vi "Dashboard Main.vi"() -> ()   [LabVIEW 2014]
uses:
  <vilib>/event_ctls.llb/eventvkey.ctl
  <vilib>/Rock Robotics/WPI/Dashboard/WPI_DashboardLogging Global.vi
  <vilib>/Rock Robotics/Network Tables/SD Write Number.vi
  <vilib>/Rock Robotics/Network Tables/SD Write Boolean.vi
  <vilib>/Rock Robotics/Network Tables/SD Read Number.vi
  <vilib>/Rock Robotics/Network Tables/SD Read Boolean.vi
  <vilib>/Rock Robotics/Network Tables/SD Write String.vi
  <vilib>/Utility/config.llb/Write Key (String).vi
  <vilib>/Utility/config.llb/Write Key (I32).vi
  <vilib>/Utility/config.llb/NI_LVConfig.lvlib
panel:
  in  "TCP":refnum<k5>
  in  "Rec Mode":enum32{"Stop", "Record", "Playback"}(radio)
  in  "Vision":u16(ring) items=["Camera Off", "USB Camera SW", "USB Camera HW", "IP Camera"]
  out "Camera IP":string
  out "Image Message":string="Timeout in Camera Communications"
  in  "Dashboard Tab":T1(tab)
  out "?":bool
  in  "Motor Saftey":bool=TRUE
  in  "Camera Settings":T2={"Frame Rate"=30, "Compression"=30, "Size"=1} {"Frame Rate" scale=1.0..30.0; "Size" items=["640x480", "320x240", "160x120"]}
  out "MotorChart R":cluster{"Numeric":dbl, "Numeric":dbl}(graph)
  out "MotorChart L":T3(graph)
  out "MotorSliders R":cluster{"MotorSlide1":dbl, "MotorSlide2":dbl} {"MotorSlide2" scale=-1.0..1.0 scale format="%#_2e"; "MotorSlide1" scale=-1.0..1.0 scale format="%#_2e"}
  out "MotorSliders L":T4 {"MotorSlide4 2" scale=0.0..14.0 scale format="%#_2e"; "MotorSlide2" scale=-1.0..1.0 scale format="%#_2e"; "MotorSlide1" scale=-1.0..1.0 scale format="%#_2e"}
  out "Gyro":dbl(knob) scale=0.0..360.0
  out "JS1 Z":dbl(slide) scale=-1.0..1.0 scale format="%#_2e"
  out "JS1 Graph":cluster{"X":dbl, "Y":dbl}[](graph)
  out "JS1 Buttons":T5
  out "JS2 Z":dbl(slide) scale=-1.0..1.0 scale format="%#_2e"
  out "JS2 Graph":cluster{"X":dbl, "Y":dbl}[](graph)
  out "JS2 Buttons":T5
  out "Mode":T6(ring)=enum."Auto Disabled"
  in  "DB Camera Config":bool
  out "fps":dbl format="%#.1g"
  out "Mbps":dbl format="%#.1g"
  out "Mbps 2":bool
  in  "DB/String 9":string
  in  "DB/String 8":string
  in  "DB/String 7":string
  in  "DB/String 6":string
  in  "DB/String 5":string
  in  "DB/String 4":string
  in  "DB/String 3":string
  in  "DB/String 2":string
  in  "DB/String 1":string
  in  "DB/String 0":string
  in  "DB/Slider 0":dbl(slide) scale=0.0..5.0
  in  "DB/Slider 1":dbl(slide) scale=0.0..5.0
  in  "DB/Slider 2":dbl(slide) scale=0.0..5.0
  in  "DB/Slider 3":dbl(slide) scale=0.0..5.0
  out "DB/LED 3":bool
  out "DB/LED 2":bool
  out "DB/LED 1":bool
  out "DB/LED 0":bool
  in  "DB/Button 3":bool
  in  "DB/Button 2":bool
  in  "DB/Button 1":bool
  in  "DB/Button 0":bool caption="New Name"
  in  "Test Slider":dbl(slide) scale=0.0..100.0 scale format="%#_3g"
  in  "On/Off":bool caption="Solenoid"
  in  "Test Name":u16(ring) items=["Select the test to run...", "Example Test", "-------------------------------", "List of tests is built in robot code.", "Replace with your own automated tests."]
  in  "Test Tree":string(tree)
  in  "Motor":cluster{"Value":dbl, "Enable":bool} {"Value" scale=-1.0..1.0 scale format="%#_3g"}
  out "Progress":T7 {"Test Progress" scale=0.0..100.0}
  in  "Rev/Fwd":cluster{"Forward":bool, "Reverse":bool}
  in  "Test Ring":u16(ring) items=["Monochrome", "Color"]
  in  "Listbox":i32(listbox)
  in  "Autonomous Program":i32(listbox)
  in  "Test System Select":enum32{"Motors", "Pneumatics"}(tab)
  in  "Test Motor Mode Select":enum32{"Encoder Mode", "Manual Mode"}(tab)
  in  "?":bool
  in  "Motor Power":dbl(knob) scale=0.0..1.0
  out "?":bool=TRUE
  out "Encoder Feedback":dbl
  in  "Encoder Setpoint":dbl
  out "Encoder RPM":dbl
  in  "?":dbl(knob) scale=-1.0..1.0
  in  "Test Action":string(combo)="Disabled"
  out "?":string="Click the top button to toggle compressor state.\nThe green button indicates if the compressor is running. If the pressure in the system is above 100psi the compressor will turn off."
  out "?":bool
  in  "?":bool
  in  "?":bool
  in  "Solenoid Action":string(combo)="Disabled"
  out "Tree":string(tree)
  out "Camera Image":T8(plugin-control)
  out "Boolean":bool
  # "Left"
  # "Front"
  # "Right"
  # "Battery"
  # "This tab is a great place for autonomous settings and robot-specific values.\nPlace controls and indicators inside this tab and match name to\nDashboard Variables on robot. You can also delete this comment."
  # "Select a system to test."
  # "Type in encoder setpoint (Ticks). Then increase the power slowly.  Encoder feedback is the traveled distance.\nThe motor should stop when staus button is green. Press reset to reset encoder."
  # "Simply drag the needle to change motor power. Motor RPM is below."
  # "Pick an action an click the button above. Double acting solenoids are automatically changed."
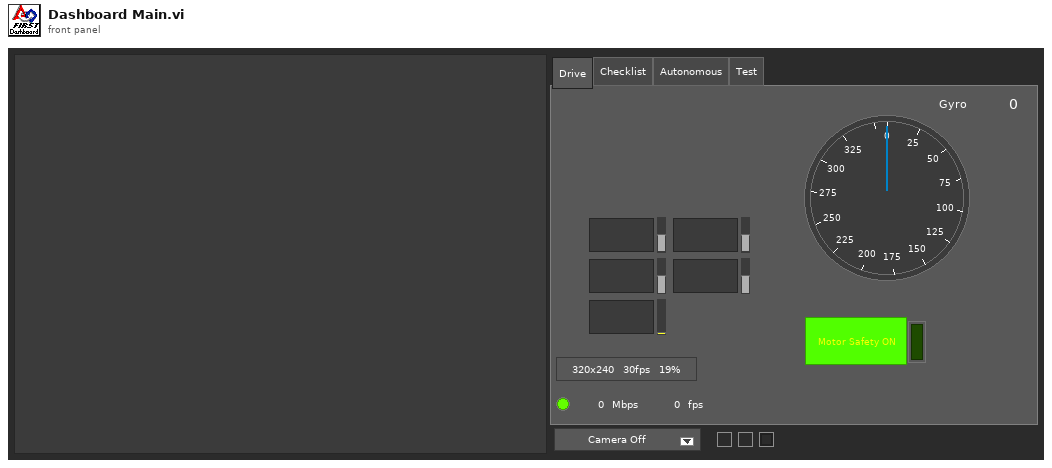
[diagram p1: front panel]
types:
  T1 = enum32{"Drive", "Basic", "Custom", "Test Var", "Checklist", "Autonomous", "Test", "Variables"}
  T2 = cluster{"Frame Rate":i32, "Compression":i32, "Size":u16}
  T3 = cluster{"Numeric":dbl, "Numeric":dbl, "Battery V":dbl}
  T4 = cluster{"MotorSlide1":dbl, "MotorSlide2":dbl, "MotorSlide4 2":dbl}
  T5 = cluster{bool, bool, bool, bool, bool, bool, bool, bool, bool, bool, bool, bool}
  T6 = enum8{"Tele-Op Disabled", "Tele-Op Enabled", "Auto Disabled", "Auto Enabled", "Test Disabled", "Test Enabled", "Disconnected", "No Code", "E-Stop"}
  T7 = cluster{"Test Progress":u8, "Test Progress Text":string}
  T8 = typedef "IMAQ Image.ctl" = refnum<image>
  T9 = enum32{"Drive", "Basic", "Custom", "Test", "Checklist", "Variables"}
  T10 = typedef "Image Type" = u32
  T11 = cluster{"Camera Image":refnum<vi>, "Dashboard Tab":refnum<vi>, "Boolean":refnum<vi>, "Vision":refnum<vi>, "Rec Mode":refnum<vi>, "Test Slider":refnum<vi>, "On/Off ":refnum<vi>, "Test Ring":refnum<vi>, "Rev/Fwd":refnum<vi>, "Test Name":refnum<vi>, "Motor":refnum<vi>, "Progress":refnum<vi>, "CheckList":refnum<vi>, "Tree":refnum<vi>, "Test Tree":refnum<vi>}
  T12 = cluster{"Error Strings":string, "Disable Counts":cluster{u16, u16}, "Rail Faults":cluster{u16, u16, u16}, "Robot IP":string, "DB Mode":u8, "Event Info":cluster{"Name":string, "Type":u8, "Number":u16, "Replay":u8}, "Camera Addr":string}
  T13 = cluster{"Storage":cluster{"Disk Free":u64, "RAM Block":u32, "RAM free":u32}, "CPU Utilization":cluster{"CPU % ISR":sgl, "CPU % Time Crit":sgl, "CPU % Timed Str":sgl, "CPU % High":sgl, "CPU % Above":sgl, "CPU % Normal":sgl, "CPU % Low":sgl}, "CAN":cluster{"% Bus Utilization":sgl, "Bus Off Cnt":u32, "TX_FIFO Full Cnt":u32, "Receive Error Cnt":u8, "Transmit Error Cnt":u8}, "HID":cluster{"HID Outputs":u32, "Rumble Low":u16, "Rumble High":u16}[]}
  T14 = cluster{"Status bits":cluster{"Test Mode":bool, "Autonomous":bool, "Enabled":bool, "Code Start":bool, "Brownout":bool, "Reserved 2":bool, "Reserved 3":bool, "E-Stop":bool}, "Code Trace":cluster{"Disabled":bool, "TeleOp":bool, "Auto":bool, "Test":bool}, "Controller Type":enum16{"unknown", "cRIO", "roboRio"}, "Code?":enum16{"unknown", "noCode", "code"}, "Battery V":dbl}
  T15 = cluster{"Control Bits":cluster{"TestMode":bool, "Autonomous":bool, "Enabled":bool, "FMS Present":bool, bool, bool, bool, "E-Stop":bool}, "Team Station ":u8, "Countdown":sgl, "Joystick Values":cluster{"Axes":dbl[], "Buttons":bool[], "POVs":i16[]}[]}
  T16 = cluster{"Axes":dbl[], "Buttons":bool[], "POVs":i16[]}[]
  T17 = cluster{"Axes":dbl[], "Buttons":bool[], "POVs":i16[]}
  T18 = cluster{"Buttons[0]":bool, "Buttons[1]":bool, "Buttons[2]":bool, "Buttons[3]":bool, "Buttons[4]":bool, "Buttons[5]":bool, "Buttons[6]":bool, "Buttons[7]":bool, "Buttons[8]":bool, "Buttons[9]":bool, "Buttons[10]":bool, "Buttons[11]":bool}
  T19 = typedef "NI_LVConfig.lvlib/Config Data RefNum.ctl" = refnum<k1>
  T20 = cluster{"Operation":enum16{"Update", "Clear"}, "Color Box":u32}[]
  T21 = typedef "eventvkey.ctl" = enum16{"ASCII", "Enter", "Return", "Shift", "Ctrl", "Alt", "Cmd", "Opt", "Caps", "NumLock", "Clear", "Break", "Up", "Down", "Left", "Right", "Insert", "Delete", "Home", "End", "PageUp", "PageDown", "Escape", "Help", "Pause", "ScrollLock", "F1", "F2", "F3", "F4", "F5", "F6", "F7", "F8", "F9", "F10", "F11", "F12", "F13", "F14", "F15", "F16", "F17", "F18", "F19", "F20", "F21", "F22", "F23", "F24", "Play", "VolumeUp", "VolumeDown", "Mute", "Two Byte Char"}
  T22 = cluster{"Image Size":bool, "Image Type":bool, "Pixel Value":bool, "ROI Information":bool, "Zoom Factor":bool}
  T23 = enum8{"Enabled", "Disabled", "Disabled and Grayed Out"}
  T24 = cluster{"Operation":enum16{"Update", "Clear"}, "Color Box":u32}
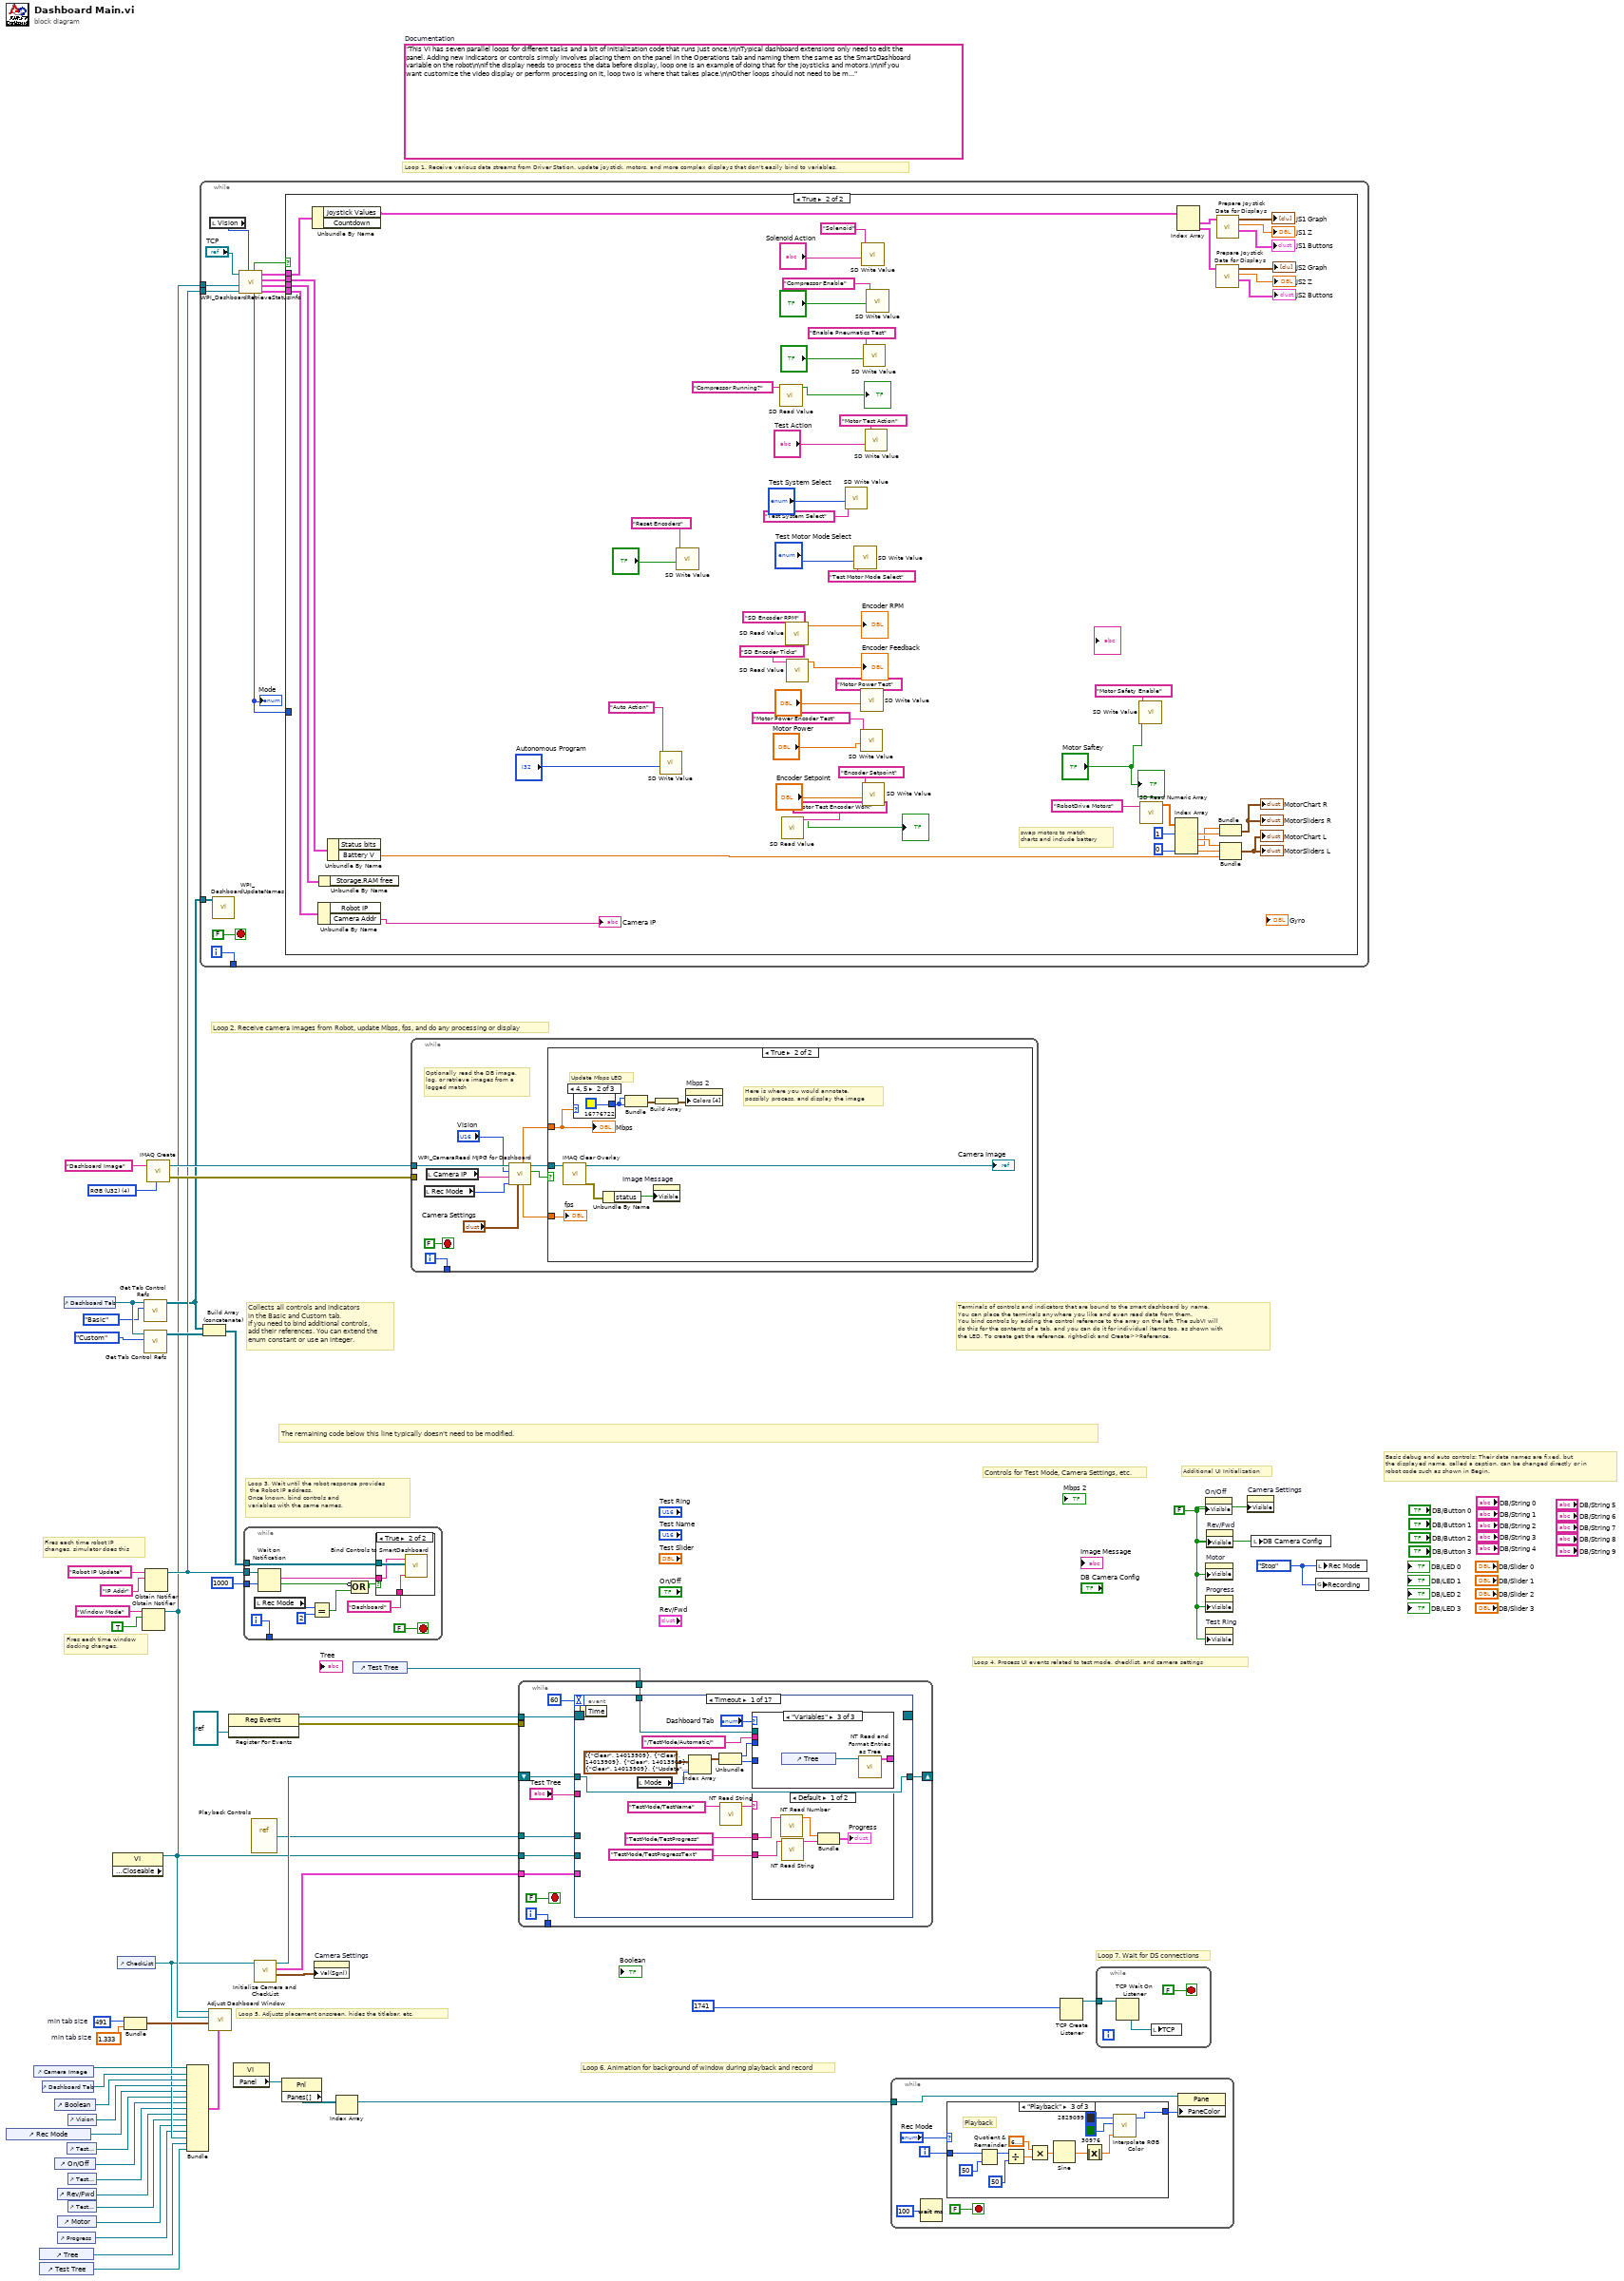
[diagram p0: block diagram]
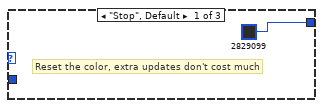
[diagram p3: hidden frame]
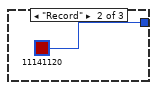
[diagram p4: hidden frame]
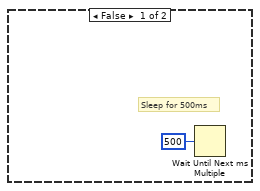
[diagram p6: hidden frame]
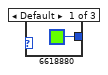
[diagram p7: hidden frame]
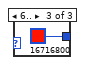
[diagram p8: hidden frame]
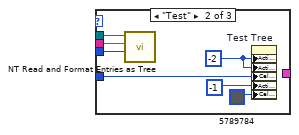
[diagram p10: hidden frame]
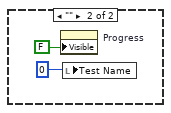
[diagram p11: hidden frame]
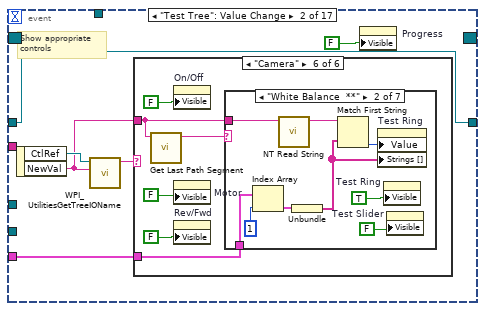
[diagram p12: hidden frame]
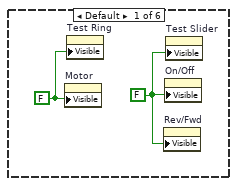
[diagram p13: hidden frame]
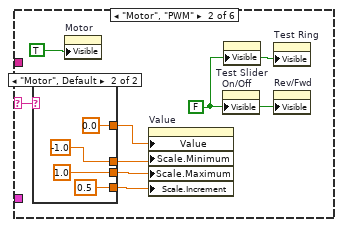
[diagram p14: hidden frame]
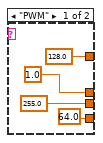
[diagram p15: hidden frame]
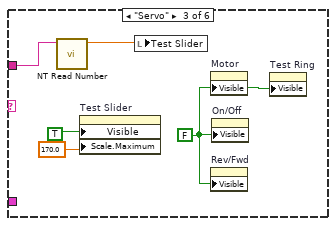
[diagram p16: hidden frame]
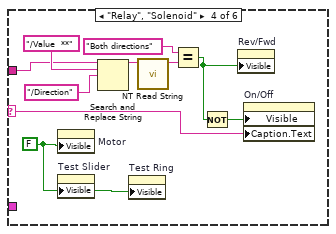
[diagram p17: hidden frame]
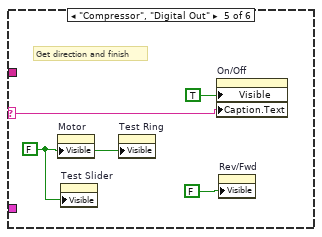
[diagram p18: hidden frame]
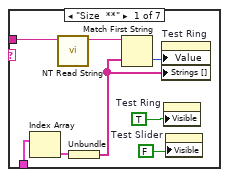
[diagram p19: hidden frame]
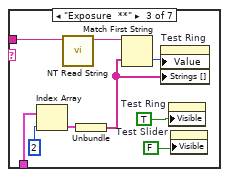
[diagram p20: hidden frame]
diagram:
  w24 = 491  # min tab size
  w23 = 1.333  # min tab size
  w32 = enum32{"Stop", "Record", "Playback"}."Stop" ("Rec Mode")
  w6 = FALSE ("Visible")
  (unwired) "This VI has seven parallel loops for different tasks and a bit of initialization code that runs just once.\n\nTypical dashboard extensions only need to edit the panel. Adding new indicators or controls simply involves placing them on the panel in the Operations tab and naming them the same as the SmartDashboard variable on the robot\n\nIf the display needs to process the data before display, loop one is an example of doing that for the joysticks and motors.\n\nIf you want customize the video display or perform processing on it, loop two is where that takes place.\n\nOther loops should not need to be modified. They are pretty standard, and document the task they perform."  # Documentation
  w52 = T10 4 items=["Grayscale (U8)", "Grayscale (I16)", "Grayscale (SGL)", "Complex (CSG)", "RGB (U32)", "HSL (U32)", "RGB (U64)"] ("Image Type")
  # "Loop 7. Wait for DS connections"
  # "Basic debug and auto controls: Their data names are fixed, but\nthe displayed name, called a caption, can be changed directly or in\nrobot code such as shown in Begin."
  # "Controls for Test Mode, Camera Settings, etc."
  # "Additional UI Initialization"
  # "Loop 6. Animation for background of window during playback and record"
  # "Fires each time robot IP\nchanges, simulator does this"
  # "Fires each time window\ndocking changes."
  # "Collects all controls and indicators\nin the Basic and Custom tab.\nIf you need to bind additional controls,\nadd their references. You can extend the\nenum constant or use an integer."
  # "The remaining code below this line typically doesn't need to be modified."
  # "Loop 4. Process UI events related to test mode, checklist, and camera settings"
  # "Terminals of controls and indicators that are bound to the smart dashboard by name.\nYou can place the terminals anywhere you like and even read data from them.\nYou bind controls by adding the control reference to the array on the left. The subVI will\ndo this for the contents of a tab, and you can do it for individual items too, as shown with\nthe LED. To create get the reference, right-click and Create>>Reference."
  # "Loop 3. Wait until the robot response provides\n the Robot IP address.\nOnce known, bind controls and\nvariables with the same names."
  # "Loop 5. Adjusts placement onscreen, hides the titlebar, etc."
  # "Loop 1. Receive various data streams from Driver Station, update joystick, motors, and more complex displays that don't easily bind to variables."
  # "Loop 2. Receive camera images from Robot, update Mbps, fps, and do any processing or display"
  n1 = control-ref of="Rec Mode"() -> (w12:refnum<vi>)
  n2 = control-ref of="Camera Image"() -> (w27:refnum<vi>)
  n3 = control-ref of="Tree"() -> (w16:refnum<vi>)
  n4 = control-ref of="Test Tree"() -> (w15:refnum<vi>)
  n5 = control-ref of="Dashboard Tab"() -> (w26:refnum<vi>)
  n6 = control-ref of="Boolean"() -> (w21:refnum<vi>)
  n7 = control-ref of="On/Off"() -> (w10:refnum<vi>)
  n8 = control-ref of="Progress"() -> (w7:refnum<vi>)
  n9 = control-ref of="Rev/Fwd"() -> (w8:refnum<vi>)
  n10 = control-ref of="Motor"() -> (w13:refnum<vi>)
  n11 = control-ref of="Dashboard Tab"() -> (w30:refnum<vi>)
  n12 = control-ref of="Test Slider"() -> (w11:refnum<vi>)
  n13 = control-ref of="Vision"() -> (w25:refnum<vi>)
  n14 = control-ref of="Test Ring"() -> (w9:refnum<vi>)
  n15 = control-ref of="Test Name"() -> (w14:refnum<vi>)
  n16 = property class="VI" props=["Front Panel.Closeable"]() -> (reference out=w31:refnum<vi>)  [unwired: 2 in, 2 out]
  n17 = control-ref of="CheckList"() -> (w17:refnum<vi>)
  n18 = Bundle("min tab size"=w24, "min tab size"=w23) -> (w22:cluster{"min tab size":i32, "min tab size":dbl})  [unwired: 1 in]
  n19 = Obtain Notifier(name (unnamed)="Window Mode", notification data type=TRUE) -> (notifier out=w3:refnum<notifier>)  [unwired: 2 in, 2 out]
  n20 = call <vilib>:"Get Tab Control Refs.vi"("Page Index"=T9."Basic" ("Dashboard Tab"), "TabControl in"=w30) -> ("ControlsOnPage"=w4:refnum<vi>[])  [unwired: 9 in]
  n21 = call <vilib>:"Get Tab Control Refs.vi"("Page Index"=T9."Custom" ("Dashboard Tab"), "TabControl in"=w30) -> ("ControlsOnPage"=w29:refnum<vi>[])  [unwired: 9 in]
  n22 = Obtain Notifier(name (unnamed)="Robot IP Update", notification data type="IP Addr" ("name (unnamed)")) -> (notifier out=w5:refnum<notifier>)  [unwired: 2 in, 2 out]
  n23 = call "IMAQ Create"("Image Name"="Dashboard Image", "Image Type"=w52) -> ("New Image"=w50:T8, "error out"=w49:errorcluster)  [unwired: 2 in, 1 out]
  n24 = Bundle("Camera Image"=w27, "Dashboard Tab"=w26, "Boolean"=w21, "Vision"=w25, "Rec Mode"=w12, "Test Slider"=w11, "On/Off"=w10, "Test Ring"=w9, "Rev/Fwd"=w8, "Test Name"=w14, "Motor"=w13, "Progress"=w7, "CheckList"=w17, "Tree"=w16, "Test Tree"=w15) -> (w18:T11)  [unwired: 1 in]
  n25 = while {
    tunnel: [w64] -> _
    tunnel: w5 -> [w58]
    tunnel: w4 -> [w57]
    tunnel: w3 -> [w53]
    i -> [w64]
    stop <- FALSE stop-if-true
    n26 = local read "Vision"() -> (w55:u16)
    n27 = call <vilib>:"WPI_DashboardUpdateNames.vi"("Controls on Tab"=w57) -> ()  [unwired: 11 in]
    n28 = call <vilib>:"WPI_DashboardRetrieveStatusInfo.vi"("Vision"=w55, "Binding Refnum"=w58, "Window Mode Notifier"=w53, "TCP Cnx"="TCP") -> ("Power and Errors"=w59:T12, "Robot Metrics"=w62:T13, "Status Info"=w63:T14, "Control Info"=w60:T15, "Robot Mode"=w56:T6, "Process?"=w61:bool)  [unwired: 2 in]
    "Mode" <- w56
    n29 = case shown="True" w61 {
      tunnel: w63 -> [_ w122]
      tunnel: w62 -> [_ w121]
      tunnel: w60 -> [_ w120]
      tunnel: w59 -> [_ w119]
      tunnel: w56 -> [_ _]
      frame False {
      }
      frame True {
        # "swap motors to match\ncharts and include battery"
        n30 = Unbundle By Name(w120) -> ("Joystick Values"=w107:T16)  [unwired: 1 out]
        n31 = Unbundle By Name(w119) -> ("Camera Addr"=→"Camera IP":string)  [unwired: 1 out]
        n32 = Unbundle By Name(w121) -> ()  [unwired: 1 out]
        n33 = Unbundle By Name(w122) -> ("Battery V"=w108:dbl)  [unwired: 1 out]
        n34 = call-poly <vilib>:"SD Write Value.vi"("Numeric"="Autonomous Program", "Name"="Auto Action") -> ()  [unwired: 8 in, 2 out]
        n35 = call-poly <vilib>:"SD Write Value.vi"("Boolean"="?", "Name"="Reset Encoders") -> ()  [unwired: 8 in, 2 out]
        n36 = call-poly <vilib>:"SD Read Value.vi"("Name"="Compressor Running?") -> ("Boolean"=→"?":bool)  [unwired: 8 in, 2 out]
        n37 = call-poly <vilib>:"SD Read Value.vi"("Name"="Motor Test Encoder Work") -> ("Boolean"=→"?":bool)  [unwired: 8 in, 2 out]
        n38 = call-poly <vilib>:"SD Read Value.vi"("Name"="SD Encoder RPM") -> ("Numeric"=→"Encoder RPM":dbl)  [unwired: 8 in, 2 out]
        n39 = call-poly <vilib>:"SD Read Value.vi"("Name"="SD Encoder Ticks") -> ("Numeric"=→"Encoder Feedback":dbl)  [unwired: 8 in, 2 out]
        n40 = call-poly <vilib>:"SD Write Value.vi"("Numeric"="Test System Select", "Name"="Test System Select") -> ()  [unwired: 8 in, 2 out]
        n41 = call-poly <vilib>:"SD Write Value.vi"("Numeric"="Test Motor Mode Select", "Name"="Test Motor Mode Select") -> ()  [unwired: 8 in, 2 out]
        n42 = call-poly <vilib>:"SD Write Value.vi"("Numeric"="Motor Power", "Name"="Motor Power Encoder Test") -> ()  [unwired: 8 in, 2 out]
        n43 = call-poly <vilib>:"SD Write Value.vi"("Numeric"="?", "Name"="Motor Power Test") -> ()  [unwired: 8 in, 2 out]
        n44 = call-poly <vilib>:"SD Write Value.vi"("String"="Solenoid Action", "Name"="Solenoid") -> ()  [unwired: 8 in, 2 out]
        n45 = call-poly <vilib>:"SD Write Value.vi"("Numeric"="Encoder Setpoint", "Name"="Encoder Setpoint") -> ()  [unwired: 8 in, 2 out]
        n46 = call-poly <vilib>:"SD Write Value.vi"("Boolean"="?", "Name"="Enable Pneumatics Test") -> ()  [unwired: 8 in, 2 out]
        n47 = call-poly <vilib>:"SD Write Value.vi"("String"="Test Action", "Name"="Motor Test Action") -> ()  [unwired: 8 in, 2 out]
        n48 = call-poly <vilib>:"SD Write Value.vi"("Boolean"="?", "Name"="Compressor Enable") -> ()  [unwired: 8 in, 2 out]
        n49 = call-poly <vilib>:"SD Write Value.vi"("Boolean"="Motor Saftey", "Name"="Motor Safety Enable") -> ()  [unwired: 8 in, 2 out]
        n50 = call <vilib>:"SD Read Numeric Array.vi"("Name"="RobotDrive Motors") -> ("Numeric Array"=w110:dbl[])  [unwired: 8 in, 2 out]
        n51 = Index Array(array=w110, index #1=1, index #4=0) -> (element #1=w114:dbl, element #2=w115:dbl, element #3=w113:dbl, element #4=w118:dbl)  [unwired: 2 in]
        n52 = Index Array(array=w107) -> (element #1=w106:T17, element #2=w101:T17)  [unwired: 2 in]
        n53 = call "Prepare Joystick Data for Displays.vi"("Joystick Values"=w101) -> ("Buttons"=→"JS2 Buttons":T18, "Z Axis"=→"JS2 Z":dbl, "Cartesian Data"=→"JS2 Graph":cluster{"X axis":dbl, "X axis":dbl}[])  [unwired: 8 in]
        n54 = call "Prepare Joystick Data for Displays.vi"("Joystick Values"=w106) -> ("Buttons"=→"JS1 Buttons":T18, "Z Axis"=→"JS1 Z":dbl, "Cartesian Data"=→"JS1 Graph":cluster{"X axis":dbl, "X axis":dbl}[])  [unwired: 8 in]
        n55 = Bundle("Numeric"=w113, "Numeric"=w114) -> (→"MotorChart R" →"MotorSliders R":cluster{"Numeric":dbl, "Numeric":dbl})  [unwired: 1 in]
        n56 = Bundle("Numeric"=w115, "Numeric"=w118, "Battery V"=w108) -> (→"MotorChart L" →"MotorSliders L":T3)  [unwired: 1 in]
        "?" <- "Motor Saftey"
      }
    }
  }
  n57 = Build Array (concatenate)(w4, w29) -> (w28:refnum<vi>[])
  n58 = call "Adjust Dashboard Window.vi"("Sizing Refnums"=w18, "Size Constraints"=w22, "VI"=w31, "Notifier in"=w3) -> ()  [unwired: 8 in]
  n59 = register-events(refnum<vi> refnum) -> (reference out=w36:refnum<event-registration>, error out=w35:errorcluster)  [unwired: 2 in]
  n60 = property class="VI"() -> ("Panel"=w39:refnum<vi>)  [unwired: 2 in, 2 out]
  n61 = while {
    tunnel: w28 -> [w134]
    tunnel: w5 -> [w132]
    tunnel: [w130] -> _
    tunnel: u32 1000 ("milliseconds to wait") -> [w129]
    i -> [w130]
    stop <- FALSE stop-if-true
    n62 = local read "Rec Mode"() -> (w125:enum32{"Stop", "Record", "Playback"})
    n63 = Wait on Notification(notifier=w132, timeout in ms (-1)=w129) -> (notification=w131:string, timed out?=w127:bool)  [unwired: 2 in, 2 out]
    n64 = Equal?(x=w125, y=u16 2 ("Rec Mode")) -> (x = y?=w126:bool)
    n65 = Compound Arithmetic op=OR(invert w127, w126) -> (w128:bool)
    n66 = case shown="True" w128 {
      tunnel: w134 -> [_ w137]
      tunnel: w131 -> [_ w136]
      tunnel: "Dashboard" -> [_ w135]
      frame False {
      }
      frame True {
        n67 = call <vilib>:"Bind Controls to SmartDashboard.vi"("Client Name"=w135, "Bound Control Refs"=w137, "Server IP Address"=w136) -> ()  [unwired: 9 in]
      }
    }
  }
  n68 = vi-ref "Playback Controls.vi"() -> (w37:refnum<vi>)
  n69 = call "Initialize Camera and CheckList.vi"("ListBox in"=w17) -> ("Cluster"=w43:cluster{"value":i32, "value":i32, "index":i32}, "Array"=w44:cluster{string[]}[], "File Refnum"=w42:T19)  [unwired: 8 in]
  n70 = property class="Pnl"(reference=w39) -> ("Panes[]"=w40:refnum<vi>[])  [unwired: 1 in, 2 out]
  n71 = property on="Camera Settings" class="Clust (strict)"("Val(Sgnl)"=w43) -> ()  [unwired: 2 in, 2 out]
  n72 = Index Array(array=w40) -> (element=w38:refnum<vi>)  [unwired: 1 in]
  n73 = control-ref of="Test Tree"() -> (w41:refnum<vi>)
  n74 = while {
    tunnel: w50 -> [w146]
    tunnel: w49 -> [_]
    tunnel: [w147] -> _
    i -> [w147]
    stop <- FALSE stop-if-true
    # "Optionally read the DB image,\nlog, or retrieve images from a\nlogged match"
    n75 = local read "Rec Mode"() -> (w140:enum32{"Stop", "Record", "Playback"})
    n76 = local read "Camera IP"() -> (w138:string)
    n77 = call <vilib>:"WPI_CameraRead MJPG for Dashboard.vi"("Camera Settings"="Camera Settings", "Rec Mode"=w140, "Camera IP"=w138, "Camera Mode"="Vision", "Refnum in"=w146) -> ("Active"=w144:bool, "Refnum out"=w145:T8, "FPS"=w143:dbl, "Bandwidth (Mbps)"=w142:dbl)  [unwired: 3 in]
    n78 = case shown="True" w144 {
      tunnel: w145 -> [_ w153]
      tunnel: w142 -> [_ w152]
      tunnel: w143 -> [_ w150]
      frame False {
        # "Sleep for 500ms"
        n79 = Wait Until Next ms Multiple(millisecond multiple=u32 500) -> ()  [unwired: 1 out]
      }
      frame True {
        # "Here is where you would annotate,\npossibly process, and display the image"
        # "Update Mbps LED"
        n80 = call "IMAQ Clear Overlay"("Image"=w153) -> ("error out"=w157:errorcluster, "Image Out"=→"Camera Image":T8)  [unwired: 2 in, 7 out]
        n81 = case shown="4, 5" w152 {
          tunnel: [u32 6618880 ("Color Box") u32 16776722 ("Color Box") u32 16716800 ("Color Box")] -> w154
          frame Default {
          }
          frame 4, 5 {
          }
          frame 6.. {
          }
        }
        n82 = Unbundle By Name(w157) -> ("status"=w158:bool)
        n83 = Bundle("Color Box"=w154, "Color Box"=w154) -> (w156:cluster{"Color Box":u32, "Color Box":u32})  [unwired: 1 out]
        n84 = property on="Image Message" class="Str"("Visible"=w158) -> ()  [unwired: 2 in, 2 out]
        n85 = Build Array(w156) -> (w155:cluster{"Color Box":u32, "Color Box":u32}[])
        n86 = property on="Mbps 2" class="Bool (strict)"("Colors [4]"=w155) -> ()  [unwired: 2 in, 2 out]
        "Mbps" <- w152
        "fps" <- w150
      }
    }
  }
  n87 = while {
    tunnel: w44 -> [w169]
    shift-right: [w168] -> _
    shift-left: w42 -> [w167]
    tunnel: [w166] -> _
    tunnel: w41 -> [w165]
    tunnel: w37 -> [w164]
    tunnel: w36 -> [w163]
    tunnel: w35 -> [_]
    tunnel: w31 -> [w162]
    i -> [w166]
    stop <- FALSE stop-if-true
    n88 = event shown="[0] Timeout" {
      selector: w163 -> [_ _ _ _ _ _ _ _ _ _ _ _ _ _ _ _ _]
      dyn-events: [_ _ _ _ _ _ _ _ _ _ _ _ _ w407 _ _ _] -> _
      timeout: u32 60 ("milliseconds to wait") -> [_ _ _ _ _ _ _ _ _ _ _ _ _ _ _ _ _]
      tunnel: w165 -> [w181 _ _ _ _ _ _ _ _ _ _ _ _ _ _ _ _]
      tunnel: "Test Tree" -> [_ _ _ _ _ _ _ _ w376 w384 w386 w390 w398 _ _ _ _]
      tunnel: w169 -> [_ w203 _ _ _ _ w340 w370 _ _ _ _ _ _ _ _ _]
      tunnel: [w177 w202 w301 w306 w314 w326 w339 w363 w375 w382 w385 w389 w397 w409 w423 w424 w434] -> w168
      tunnel: w167 -> [w177 w202 w301 w306 w314 w326 w338 w363 w375 w382 w385 w389 w397 w409 w423 w424 w434]
      tunnel: w164 -> [_ _ _ _ _ _ _ _ _ _ _ _ _ w410 _ w427 _]
      tunnel: w162 -> [_ _ _ _ _ _ _ _ _ _ _ _ _ w405 _ _ _]
      event Timeout {
        n89 = event-data() -> ()  [unwired: 1 in, 1 out]
        n90 = local read "Mode"() -> (w180:T6)
        n91 = Index Array(array=T20 [{"Operation"=enum."Clear", "Color Box"=14013909}, {"Operation"=enum."Clear", "Color Box"=14013909}, {"Operation"=enum."Clear", "Color Box"=14013909}, {"Operation"=enum."Clear", "Color Box"=14013909}, {"Operation"=enum."Update", "Color Box"=14013909}, {"Operation"=enum."Update", "Color Box"=16777215}, {"Operation"=enum."Clear", "Color Box"=14013909}, {"Operation"=enum."Clear", "Color Box"=14013909}, {"Operation"=enum."Clear", "Color Box"=14013909}], index=w180) -> (element=w175:T24)
        n92 = Unbundle(w175) -> ("Operation"=w174:enum16{"Update", "Clear"}, "Color Box"=w173:u32)
        n93 = call <vilib>:"NT Read String.vi"("Name"="TestMode/TestName") -> ("String"=w184:string)  [unwired: 9 in, 1 out]
        n94 = case shown="\"Variables\"" "Dashboard Tab" {
          tunnel: w181 -> [_ w192 _]
          tunnel: "/TestMode/Automatic/" ("Name Pattern") -> [_ w191 _]
          tunnel: w174 -> [_ w190 _]
          tunnel: [_ _ w194] -> _
          tunnel: w173 -> [_ w186 _]
          frame "Custom", Default {
          }
          frame "Test" {
            w189 = -2 ("Active Item:Row Number")
            n95 = call <vilib>:"NT Read and Format Entries as Tree.vi"("Operation"=w190, "Name Pattern"=w191, "Tree Refnum"=w192) -> ()  [unwired: 7 in, 2 out]
            n96 = property on="Test Tree" class="Tree (strict)"("Active Item Row Number"=w189, "ActiveColNum"=w189, "CellBG"=w186, "Active Item Row Number"=-1 ("Active Item:Row Number"), "CellBG"=u32 5789784 ("Color Box")) -> ()  [unwired: 2 in, 2 out]
          }
          frame "Variables" {
            n97 = control-ref of="Tree"() -> (w193:refnum<vi>)
            n98 = call <vilib>:"NT Read and Format Entries as Tree.vi"("Tree Refnum"=w193) -> ("Formatted Strings"=w194:cluster{"Name":string, "Value":string}[])  [unwired: 9 in, 1 out]
          }
        }
        n99 = case shown="Default" w184 {
          tunnel: "TestMode/TestProgress" ("Name") -> [w196 _]
          tunnel: "TestMode/TestProgressText" ("Name") -> [w195 _]
          frame Default {
            n100 = call <vilib>:"NT Read Number.vi"("Name"=w196) -> ("Numeric"=w197:dbl)  [unwired: 9 in, 1 out]
            n101 = call <vilib>:"NT Read String.vi"("Name"=w195) -> ("String"=w198:string)  [unwired: 9 in, 1 out]
            n102 = Bundle("Numeric"=w197, "String"=w198) -> (→"Progress":cluster{"Numeric":dbl, "String":string})  [unwired: 1 in]
          }
          frame "" {
            n103 = property on="Progress" class="Clust (strict)"("Visible"=FALSE) -> ()  [unwired: 2 in, 2 out]
            n104 = local write "Test Name"(u16 0) -> ()
          }
        }
      }
      event "Test Tree": Value Change {
        # "Show appropriate\ncontrols"
        n105 = event-data() -> ("CtlRef"=w206:refnum<vi>, "NewVal"=w204:string)  [unwired: 1 in]
        n106 = call <vilib>:"WPI_UtilitiesGetTreeIOName.vi"("NewVal"=w204, "TreeControl in"=w206) -> ("I/O Name"=w207:string)  [unwired: 9 in]
        n107 = case shown="\"Camera\"" w207 {
          selector: w207 -> [_ w214 _ w232 w241 _]
          tunnel: w204 -> [_ _ w229 w231 _ w248]
          tunnel: w203 -> [_ _ _ _ _ w247]
          frame Default {
            w209 = FALSE ("Visible")
            w208 = FALSE ("Visible")
            n108 = property on="Motor" class="Clust (strict)"("Visible"=w208) -> ()  [unwired: 2 in, 2 out]
            n109 = property on="Test Ring" class="Ring (strict)"("Visible"=w208) -> ()  [unwired: 2 in, 2 out]
            n110 = property on="Rev/Fwd" class="Clust (strict)"("Visible"=w209) -> ()  [unwired: 2 in, 2 out]
            n111 = property on="On/Off" class="Bool (strict)"("Visible"=w209) -> ()  [unwired: 2 in, 2 out]
            n112 = property on="Test Slider" class="Slide (strict)"("Visible"=w209) -> ()  [unwired: 2 in, 2 out]
          }
          frame "Motor", "PWM" {
            w215 = FALSE ("Visible")
            n113 = case shown="\"Motor\", Default" w214 {
              tunnel: [1.0 ("Value") -1.0 ("Value")] -> w213
              tunnel: [255.0 ("Value") 1.0 ("Value")] -> w212
              tunnel: [128.0 ("Value") 0.0 ("Value")] -> w211
              tunnel: [64.0 ("Value") 0.5 ("Value")] -> w210
              frame "PWM" {
              }
              frame "Motor", Default {
              }
            }
            n114 = property on="Motor" class="Clust (strict)"("Visible"=TRUE) -> ()  [unwired: 2 in, 2 out]
            n115 = property on="Value" class="Slide (strict)"("Value"=w211, "Scale.Minimum"=w213, "Scale.Maximum"=w212, "Scale.Increment"=w210) -> ()  [unwired: 2 in, 2 out]
            n116 = property on="On/Off" class="Bool (strict)"("Visible"=w215) -> ()  [unwired: 2 in, 2 out]
            n117 = property on="Test Slider" class="Slide (strict)"("Visible"=w215) -> ()  [unwired: 2 in, 2 out]
            n118 = property on="Test Ring" class="Ring (strict)"("Visible"=w215) -> ()  [unwired: 2 in, 2 out]
            n119 = property on="Rev/Fwd" class="Clust (strict)"("Visible"=w215) -> ()  [unwired: 2 in, 2 out]
          }
          frame "Servo" {
            w227 = FALSE ("Visible")
            n120 = call <vilib>:"NT Read Number.vi"("Name"=w229) -> ("Numeric"=w228:dbl)  [unwired: 9 in, 1 out]
            n121 = property on="Test Slider" class="Slide (strict)"("Visible"=TRUE, "Scale.Maximum"=170.0 ("Scale.Range:Maximum")) -> ()  [unwired: 2 in, 2 out]
            n122 = local write "Test Slider"(w228) -> ()
            n123 = property on="Motor" class="Clust (strict)"("Visible"=w227) -> ()  [unwired: 2 in, 2 out]
            n124 = property on="Rev/Fwd" class="Clust (strict)"("Visible"=w227) -> ()  [unwired: 2 in, 2 out]
            n125 = property on="On/Off" class="Bool (strict)"("Visible"=w227) -> ()  [unwired: 2 in, 2 out]
            n126 = property on="Test Ring" class="Ring (strict)"("Visible"=w227) -> ()  [unwired: 2 in, 2 out]
          }
          frame "Relay", "Solenoid" {
            w230 = FALSE ("Visible")
            n127 = property on="Motor" class="Clust (strict)"("Visible"=w230) -> ()  [unwired: 2 in, 2 out]
            n128 = property on="Test Slider" class="Slide (strict)"("Visible"=w230) -> ()  [unwired: 2 in, 2 out]
            n129 = Search and Replace String(input string=w231, search string="/Value  **", replace string="/Direction") -> (result string=w237:string)  [unwired: 5 in, 3 out]
            n130 = property on="Test Ring" class="Ring (strict)"("Visible"=w230) -> ()  [unwired: 2 in, 2 out]
            n131 = call <vilib>:"NT Read String.vi"("Name"=w237) -> ("String"=w235:string)  [unwired: 9 in, 1 out]
            n132 = Equal?(x="Both directions", y=w235) -> (x = y?=w233:bool)
            n133 = Not(x=w233) -> (.not. x?=w234:bool)
            n134 = property on="Rev/Fwd" class="Clust (strict)"("Visible"=w233) -> ()  [unwired: 2 in, 2 out]
            n135 = property on="On/Off" class="Bool (strict)"("Visible"=w234, "Caption.Text"=w232) -> ()  [unwired: 2 in, 2 out]
          }
          frame "Compressor", "Digital Out" {
            w240 = FALSE ("Visible")
            # "Get direction and finish"
            n136 = property on="Motor" class="Clust (strict)"("Visible"=w240) -> ()  [unwired: 2 in, 2 out]
            n137 = property on="Test Slider" class="Slide (strict)"("Visible"=w240) -> ()  [unwired: 2 in, 2 out]
            n138 = property on="Test Ring" class="Ring (strict)"("Visible"=w240) -> ()  [unwired: 2 in, 2 out]
            n139 = property on="On/Off" class="Bool (strict)"("Visible"=TRUE, "Caption.Text"=w241) -> ()  [unwired: 2 in, 2 out]
            n140 = property on="Rev/Fwd" class="Clust (strict)"("Visible"=FALSE) -> ()  [unwired: 2 in, 2 out]
          }
          frame "Camera" {
            n141 = call <vilib>:"Get Last Path Segment.vi"("String in"=w248) -> ("String out"=w249:string)  [unwired: 10 in]
            n142 = property on="On/Off" class="Bool (strict)"("Visible"=FALSE) -> ()  [unwired: 2 in, 2 out]
            n143 = property on="Motor" class="Clust (strict)"("Visible"=FALSE) -> ()  [unwired: 2 in, 2 out]
            n144 = property on="Rev/Fwd" class="Clust (strict)"("Visible"=FALSE) -> ()  [unwired: 2 in, 2 out]
            n145 = case shown="\"White Balance  **\"" w249 {
              tunnel: w248 -> [w255 w264 w273 w282 w291 _ w297]
              tunnel: w247 -> [w253 w261 w270 w279 w288 _ _]
              frame "Size  **" {
                n146 = Index Array(array=w253) -> (element=w252:cluster{string[]})  [unwired: 1 in]
                n147 = call <vilib>:"NT Read String.vi"("Name"=w255) -> ("String"=w254:string)  [unwired: 9 in, 1 out]
                n148 = Unbundle(w252) -> (w250:string[])
                n149 = Match First String(2:w250, 3:w254) -> (0:w251:i32)  [unwired: 1 out]
                n150 = property on="Test Ring" class="Ring (strict)"("Value"=w251, "Strings []"=w250) -> ()  [unwired: 2 in, 2 out]
                n151 = property on="Test Ring" class="Ring (strict)"("Visible"=TRUE) -> ()  [unwired: 2 in, 2 out]
                n152 = property on="Test Slider" class="Slide (strict)"("Visible"=FALSE) -> ()  [unwired: 2 in, 2 out]
              }
              frame "White Balance  **" {
                n153 = Index Array(array=w261, index=1) -> (element=w262:cluster{string[]})
                n154 = call <vilib>:"NT Read String.vi"("Name"=w264) -> ("String"=w263:string)  [unwired: 9 in, 1 out]
                n155 = Unbundle(w262) -> (w259:string[])
                n156 = Match First String(2:w259, 3:w263) -> (0:w258:i32)  [unwired: 1 out]
                n157 = property on="Test Ring" class="Ring (strict)"("Value"=w258, "Strings []"=w259) -> ()  [unwired: 2 in, 2 out]
                n158 = property on="Test Ring" class="Ring (strict)"("Visible"=TRUE) -> ()  [unwired: 2 in, 2 out]
                n159 = property on="Test Slider" class="Slide (strict)"("Visible"=FALSE) -> ()  [unwired: 2 in, 2 out]
              }
              frame "Exposure  **" {
                n160 = Index Array(array=w270, index=2) -> (element=w271:cluster{string[]})
                n161 = call <vilib>:"NT Read String.vi"("Name"=w273) -> ("String"=w272:string)  [unwired: 9 in, 1 out]
                n162 = Unbundle(w271) -> (w267:string[])
                n163 = Match First String(2:w267, 3:w272) -> (0:w268:i32)  [unwired: 1 out]
                n164 = property on="Test Ring" class="Ring (strict)"("Value"=w268, "Strings []"=w267) -> ()  [unwired: 2 in, 2 out]
                n165 = property on="Test Ring" class="Ring (strict)"("Visible"=TRUE) -> ()  [unwired: 2 in, 2 out]
                n166 = property on="Test Slider" class="Slide (strict)"("Visible"=FALSE) -> ()  [unwired: 2 in, 2 out]
              }
              frame "Exposure Priority  **" {
                n167 = Index Array(array=w279, index=3) -> (element=w280:cluster{string[]})
                n168 = call <vilib>:"NT Read String.vi"("Name"=w282) -> ("String"=w281:string)  [unwired: 9 in, 1 out]
                n169 = Unbundle(w280) -> (w276:string[])
                n170 = Match First String(2:w276, 3:w281) -> (0:w277:i32)  [unwired: 1 out]
                n171 = property on="Test Ring" class="Ring (strict)"("Value"=w277, "Strings []"=w276) -> ()  [unwired: 2 in, 2 out]
                n172 = property on="Test Ring" class="Ring (strict)"("Visible"=TRUE) -> ()  [unwired: 2 in, 2 out]
                n173 = property on="Test Slider" class="Slide (strict)"("Visible"=FALSE) -> ()  [unwired: 2 in, 2 out]
              }
              frame "Color Enable  **" {
                n174 = Index Array(array=w288, index=4) -> (element=w289:cluster{string[]})
                n175 = call <vilib>:"NT Read String.vi"("Name"=w291) -> ("String"=w290:string)  [unwired: 9 in, 1 out]
                n176 = Unbundle(w289) -> (w285:string[])
                n177 = Match First String(2:w285, 3:w290) -> (0:w286:i32)  [unwired: 1 out]
                n178 = property on="Test Ring" class="Ring (strict)"("Value"=w286, "Strings []"=w285) -> ()  [unwired: 2 in, 2 out]
                n179 = property on="Test Ring" class="Ring (strict)"("Visible"=TRUE) -> ()  [unwired: 2 in, 2 out]
                n180 = property on="Test Slider" class="Slide (strict)"("Visible"=FALSE) -> ()  [unwired: 2 in, 2 out]
              }
              frame Default {
                n181 = property on="Test Ring" class="Ring (strict)"("Visible"=FALSE) -> ()  [unwired: 2 in, 2 out]
                n182 = property on="Test Slider" class="Slide (strict)"("Visible"=FALSE) -> ()  [unwired: 2 in, 2 out]
              }
              frame "Brightness  **", "Color Level  **", "Compression  **", "FPS  **", "Sharpness  **" {
                n183 = call <vilib>:"NT Read Number.vi"("Name"=w297) -> ("Numeric"=w296:dbl)  [unwired: 9 in, 1 out]
                n184 = local write "Test Slider"(w296) -> ()
                n185 = property on="Test Ring" class="Ring (strict)"("Visible"=FALSE) -> ()  [unwired: 2 in, 2 out]
                n186 = property on="Test Slider" class="Slide (strict)"("Visible"=TRUE, "Scale.Maximum"=100.0 ("Scale.Range:Maximum")) -> ()  [unwired: 2 in, 2 out]
              }
            }
          }
        }
        n187 = property on="Progress" class="Clust (strict)"("Visible"=FALSE) -> ()  [unwired: 2 in, 2 out]
      }
      event "Test Name": Mouse Enter {
        # "Populate the ring with the list of tests"
        n188 = event-data() -> ()  [unwired: 1 in, 1 out]
        n189 = call <vilib>:"NT Read String Array.vi"("Name"="TestMode/TestList") -> ("String Array"=w305:string[])  [unwired: 9 in, 1 out]
        n190 = Build Array (concatenate)("Select the test to run...", w305) -> (w304:string[])
        n191 = property on="Test Name" class="Ring (strict)"("Strings []"=w304) -> ()  [unwired: 2 in, 2 out]
      }
      event "Test Name": Value Change {
        w307 = FALSE ("Visible")
        # "Tell the robot the test name to run"
        n192 = event-data() -> ("NewVal"=w311:u16)  [unwired: 1 in]
        n193 = property on="Test Name" class="Ring (strict)"() -> ("Strings []"=w312:string[])  [unwired: 2 in, 2 out]
        n194 = local write "Progress"(T7 {"Test Progress"=0, "Test Progress Text"=""} ("Progress")) -> ()
        n195 = Index Array(array=w312, index=w311) -> (element=w310:string)
        n196 = call <vilib>:"NT Write String.vi"("String"=w310, "Name"="TestMode/TestName") -> ()  [unwired: 9 in, 1 out]
        n197 = property on="Progress" class="Clust (strict)"("Visible"=TRUE) -> ()  [unwired: 2 in, 2 out]
        n198 = property on="Motor" class="Clust (strict)"("Visible"=w307) -> ()  [unwired: 2 in, 2 out]
        n199 = property on="Test Slider" class="Slide (strict)"("Visible"=w307) -> ()  [unwired: 2 in, 2 out]
        n200 = property on="On/Off" class="Bool (strict)"("Visible"=w307) -> ()  [unwired: 2 in, 2 out]
        n201 = property on="Rev/Fwd" class="Clust (strict)"("Visible"=w307) -> ()  [unwired: 2 in, 2 out]
        n202 = property on="Test Ring" class="Ring (strict)"("Visible"=w307) -> ()  [unwired: 2 in, 2 out]
      }
      event "Listbox": Double Click {
        # "Shift clears all"
        # "Update symbols on the listbox"
        n203 = event-data() -> ("PlatMods.Shift"=w315:bool, "Row"=w317:i32)  [unwired: 1 in]
        n204 = case shown="True" w315 {
          tunnel: w317 -> [w321 _]
          tunnel: 1 -> [w320 _]
          frame False {
            n205 = property on="Listbox" class="LstBox (strict)"() -> ("Item Symbols"=w319:i32[])  [unwired: 2 in, 2 out]
            n206 = Replace Array Subset(array=w319, new element=w320, index=w321) -> (w318:i32[])
            n207 = property on="Listbox" class="LstBox (strict)"("Item Symbols"=w318) -> ()  [unwired: 2 in, 2 out]
          }
          frame True {
            w322 = 0 ("Top Row")
            n208 = property on="Listbox" class="LstBox (strict)"() -> ("Number of Rows"=w324:u32)  [unwired: 2 in, 2 out]
            n209 = Initialize Array(0, w324) -> (w323:i32[])
            n210 = property on="Listbox" class="LstBox (strict)"("Top Row"=w322, "Value"=w322, "Item Symbols"=w323) -> ()  [unwired: 2 in, 2 out]
          }
        }
      }
      event "Listbox": Key Down {
        # "Update symbols on the listbox\nLeft and right keys check and uncheck"
        n211 = event-data() -> ("VKey"=w328:T21)  [unwired: 1 in]
        n212 = case shown="\"Left\", \"Right\"" w328 {
          selector: w328 -> [w333 _]
          tunnel: eventvkey."Left" ("VKey") -> [w331 _]
          frame "Left", "Right" {
            n213 = Equal?(x=w331, y=w333) -> (x = y?=w332:bool)
            n214 = Select(t=0, s=w332, f=1) -> (s? t:f=w334:i32)
            n215 = property on="Listbox" class="LstBox (strict)"() -> ("Item Symbols"=w337:i32[])  [unwired: 2 in, 2 out]
            n216 = Replace Array Subset(array=w337, new element=w334, index="Listbox") -> (w336:i32[])
            n217 = property on="Listbox" class="LstBox (strict)"("Item Symbols"=w336) -> ()  [unwired: 2 in, 2 out]
          }
          frame Default {
          }
        }
      }
      event "DB Camera Config": Value Change {
        # "Show or hide the cluster of controls, store in ini file"
        n218 = event-data() -> ("NewVal"=w341:bool)  [unwired: 1 in]
        n219 = case shown="False" w341 {
          tunnel: w340 -> [w350 _]
          tunnel: [w343 w361] -> w339
          tunnel: w338 -> [w342 w361]
          frame False {
            w357 = "Camera"
            w360 = FALSE ("Visible")
            n220 = local read "Camera Settings"() -> (w349:T2)
            n221 = Index Array(array=w350) -> (element=w353:cluster{string[]})  [unwired: 1 in]
            n222 = Unbundle(w349) -> ("Frame Rate"=w348:i32, "Compression"=w347:i32, "Size"=w351:u16)
            n223 = Unbundle(w353) -> (w352:string[])
            n224 = Index Array(array=w352, index=w351) -> (element=w346:string)
            n225 = call-poly <vilib>:"Write Key.vi"("section"=w357, "value"=w346, "key"="Size", "refnum"=w342) -> ("refnum out"=w359:T19)  [unwired: 2 in, 5 out]
            n226 = call-poly <vilib>:"Write Key.vi"("section"=w357, "value"=w348, "key"="FrameRate", "refnum"=w359) -> ("refnum out"=w358:T19)  [unwired: 1 in, 6 out]
            n227 = property on="Camera Settings" class="Clust (strict)"("Visible"=w360) -> ()  [unwired: 2 in, 2 out]
            n228 = local write "DB Camera Config"(w360) -> ()
            n229 = call-poly <vilib>:"Write Key.vi"("section"=w357, "value"=w347, "key"="Compression", "refnum"=w358) -> ("refnum out"=w344:T19)  [unwired: 1 in, 6 out]
            n230 = call <vilib>:"Close Config Data.vi"("refnum"=w344) -> ("file path"=w345:path)  [unwired: 2 in, 8 out]
            n231 = call <vilib>:"Open Config Data.vi"("configuration file path"=w345) -> ("refnum"=w343:T19)  [unwired: 8 in, 2 out]
          }
          frame True {
            n232 = property on="Camera Settings" class="Clust (strict)"("Visible"=TRUE) -> ()  [unwired: 2 in, 2 out]
          }
        }
      }
      event "Camera Settings": Value Change {
        # "Update summary string when any elements of DB camera change"
        n233 = event-data() -> ("NewVal"=w374:T2)  [unwired: 1 in]
        n234 = Index Array(array=w370) -> (element=w369:cluster{string[]})  [unwired: 1 in]
        n235 = Unbundle(w374) -> ("Frame Rate"=w365:i32, "Compression"=w364:i32, "Size"=w367:u16)
        n236 = Unbundle(w369) -> (w368:string[])
        n237 = Index Array(array=w368, index=w367) -> (element=w366:string)
        n238 = Format Into String(format string="%s   %dfps   %d%%", w366, w365, w364) -> (resulting string=w371:string)  [unwired: 2 in, 1 out]
        n239 = Build Array(w371) -> (w372:string[])
        n240 = property on="DB Camera Config" class="Bool (strict)"("Strings [4]"=w372) -> ()  [unwired: 2 in, 2 out]
      }
      event "Motor.Enable": Value Change {
        # "When the test mode otor enable helper is set, update that\ntree row item's value"
        n241 = event-data() -> ("NewVal"=w380:bool)  [unwired: 1 in]
        n242 = Unbundle("Motor") -> ("Value"=w379:dbl)  [unwired: 1 out]
        n243 = Select(t=w379, s=w380, f=0.0) -> (s? t:f=w377:dbl)
        n244 = call <vilib>:"NT Write Number.vi"("Numeric"=w377, "Name"=w376) -> ()  [unwired: 9 in, 1 out]
      }
      event "Test Slider": Value Change {
        # "When the test mode slider helper is set, update that\ntree row item's value"
        n245 = event-data() -> ("NewVal"=w383:dbl)  [unwired: 1 in]
        n246 = call <vilib>:"NT Write Number.vi"("Numeric"=w383, "Name"=w384) -> ()  [unwired: 9 in, 1 out]
      }
      event "On/Off": Value Change {
        # "When the test mode on/off helper value is set, update that\ntree row item's value"
        n247 = event-data() -> ("NewVal"=w388:bool)  [unwired: 1 in]
        n248 = Boolean To (0,1)(Boolean=w388) -> (0, 1=w387:i16)
        n249 = call <vilib>:"NT Write Number.vi"("Numeric"=w387, "Name"=w386) -> ()  [unwired: 9 in, 1 out]
      }
      event "Rev/Fwd": Value Change {
        # "When the test mode helper value for relays is set, update that\ntree row item's value"
        n250 = event-data() -> ("NewVal.Forward"=w396:bool, "NewVal.Reverse"=w395:bool)  [unwired: 1 in]
        n251 = Boolean To (0,1)(Boolean=w396) -> (0, 1=w392:i16)
        n252 = Boolean To (0,1)(Boolean=w395) -> (0, 1=w394:i16)
        n253 = Negate(x=w394) -> (-x=w393:i16)
        n254 = Add(x=w392, y=w393) -> (x+y=w391:i16)
        n255 = call <vilib>:"NT Write Number.vi"("Numeric"=w391, "Name"=w390) -> ()  [unwired: 9 in, 1 out]
      }
      event "Test Ring": Value Change {
        # "When a test mode helper value is selected from the ring,\nset the tree item's variable to the string value"
        n256 = event-data() -> ("NewVal"=w400:u16)  [unwired: 1 in]
        n257 = property on="Test Ring" class="Ring (strict)"() -> ("Strings []"=w401:string[])  [unwired: 2 in, 2 out]
        n258 = Index Array(array=w401, index=w400) -> (element=w399:string)
        n259 = call <vilib>:"NT Write String.vi"("String"=w399, "Name"=w398) -> ()  [unwired: 9 in, 1 out]
      }
      event "Rec Mode": Value Change {
        # "Update globals for recording mode and path to read log from.\nClear when logging and let NetworkTables set path for vision to\nuse."
        n260 = event-data() -> ("NewVal"=w411:enum32{"Stop", "Record", "Playback"})  [unwired: 1 in]
        n261 = case shown="\"Playback\"" w411 {
          tunnel: w410 -> [_ w413 w421]
          tunnel: [_ _ w420] -> w407
          tunnel: [_ _ w419] -> _
          tunnel: w405 -> [_ _ w417]
          tunnel: cluster{i32, i32} {-250, 170} -> [_ _ w416]
          tunnel: [_ _ T22 {"Image Size"=TRUE, "Image Type"=TRUE, "Pixel Value"=TRUE, "ROI Information"=TRUE, "Zoom Factor"=FALSE} ("Image Information Shown:All Elements")] -> w403
          tunnel: [_ _ TRUE ("Zoom Factor")] -> w402
          frame Default {
          }
          frame "Stop", "Record" {
            # "Place Window too"
            n262 = invoke class="VI" method="FP.Close"(reference=w413) -> (reference out=w412:refnum<vi>)  [unwired: 2 in, 2 out]
            n263 = invoke class="VI" method="Abort VI"(reference=w412) -> ()  [unwired: 2 in, 3 out]
          }
          frame "Playback" {
            n264 = call "Open Playback Panel.vi"("Offset"=w416, "DB VI Ref"=w417, "Playback in"=w421) -> ("Playback out"=w418:refnum<vi>)  [unwired: 8 in]
            n265 = register-events(w418) -> (reference out=w420:refnum<event-registration>, error out=w419:errorcluster)  [unwired: 2 in]
          }
        }
        n266 = global write "WPI_DashboardLogging Global.vi" "Recording"(w411) -> ()
        n267 = global write "WPI_DashboardLogging Global.vi" "Logging Filename"(path "") -> ()
        n268 = property on="Camera Image" class="ImageControl"("Image Information Shown"=w403, "Image Information Visible"=w402) -> ()  [unwired: 2 in, 2 out]
        n269 = call <vilib>:"WPI_DashboardNT Log FieldName Cache.vi"("Operation"=enum16{"Lookup/Add", "Index", "Clear"}."Clear") -> ()  [unwired: 8 in, 3 out]
      }
      event Panel Close {
        w422 = enum32{"Stop", "Record", "Playback"}."Stop" ("Rec Mode")
        # "Playback window has been closed, abort"
        n270 = event-data() -> ()  [unwired: 1 in, 4 out]
        n271 = local write "Rec Mode"(w422) -> ()
        n272 = global write "WPI_DashboardLogging Global.vi" "Recording"(w422) -> ()
      }
      event Panel Close {
        # "Abort playback window and ourself"
        n273 = event-data() -> ()  [unwired: 1 in, 4 out]
        n274 = invoke class="VI" method="FP.Close"(reference=w427) -> (reference out=w426:refnum<vi>)  [unwired: 2 in, 2 out]
        n275 = invoke class="VI" method="Abort VI"(reference=w426) -> (error out=w425:errorcluster)  [unwired: 2 in, 2 out]
        n276 = invoke class="VI" method="Abort VI"(error in=w425) -> ()  [unwired: 2 in, 3 out]
      }
      event "Vision": Value Change {
        # "Enable/Disable Compression slider.\nHW USB is hard-coded into the camera"
        n277 = event-data() -> ("NewVal"=w433:u16)  [unwired: 1 in]
        n278 = Equal?(x=w433, y=u32 2 ("milliseconds to wait")) -> (x = y?=w431:bool)
        n279 = Select(t=T23."Disabled and Grayed Out" ("Disabled"), s=w431, f=T23."Enabled" ("Disabled")) -> (s? t:f=w428:T23)
        n280 = property on="Compression" class="Slide (strict)"("DisabledEnum"=w428) -> ()  [unwired: 2 in, 2 out]
      }
    }
  }
  n281 = while {
    tunnel: w38 -> [w436]
    i -> [w439]
    stop <- FALSE stop-if-true
    n282 = Wait (ms)(milliseconds to wait=u32 100) -> ()  [unwired: 1 out]
    n283 = case shown="\"Playback\"" "Rec Mode" {
      tunnel: w439 -> [_ _ w454]
      tunnel: [u32 2829099 ("Base Color") u32 11141120 ("Target Color") w443] -> w435
      frame "Stop", Default {
        # "Reset the color, extra updates don't cost much"
      }
      frame "Record" {
      }
      frame "Playback" {
        # "Playback"
        n284 = Quotient & Remainder(x=w454, y=u32 50 ("milliseconds to wait")) -> (x-y*floor(x/y)=w450:u32)  [unwired: 1 out]
        n285 = Divide(x=w450, y=u32 50 ("milliseconds to wait")) -> (x/y=w447:dbl)
        n286 = Multiply(x=6.283185307179586, y=w447) -> (x*y=w452:dbl)
        n287 = Sine(x=w452) -> (sin(x)=w451:dbl)
        n288 = Absolute Value(x=w451) -> (abs(x)=w444:dbl)
        n289 = call "Interpolate RGB Color.vi"("Proportion"=w444, "Target Color"=u32 30976, "Base Color"=u32 2829099) -> ("Result Color"=w443:u32)  [unwired: 8 in]
      }
    }
    n290 = property class="Pane"(reference=w436, "PaneColor"=w435) -> ()  [unwired: 1 in, 2 out]
  }
  n291 = TCP Create Listener(10:u16 1741 ("timeout ms (25000)")) -> (3:w1:refnum<k5>)  [unwired: 4 in, 2 out]
  n292 = while {
    tunnel: w1 -> [w456]
    stop <- FALSE stop-if-true
    n293 = TCP Wait On Listener(11:w456) -> (4:w455:refnum<k5>)  [unwired: 3 in, 4 out]
    n294 = local write "TCP"(w455) -> ()
  }
  n295 = property on="On/Off" class="Bool (strict)"("Visible"=w6) -> ()  [unwired: 2 in, 2 out]
  n296 = property on="Motor" class="Clust (strict)"("Visible"=w6) -> ()  [unwired: 2 in, 2 out]
  n297 = property on="Progress" class="Clust (strict)"("Visible"=w6) -> ()  [unwired: 2 in, 2 out]
  n298 = property on="Test Ring" class="Ring (strict)"("Visible"=w6) -> ()  [unwired: 2 in, 2 out]
  n299 = property on="Rev/Fwd" class="Clust (strict)"("Visible"=w6) -> ()  [unwired: 2 in, 2 out]
  n300 = property on="Camera Settings" class="Clust (strict)"("Visible"=w6) -> ()  [unwired: 2 in, 2 out]
  n301 = local write "DB Camera Config"(w6) -> ()
  n302 = global write "WPI_DashboardLogging Global.vi" "Recording"(w32) -> ()
  n303 = local write "Rec Mode"(w32) -> ()
